vi "Untitled 2.vi"() -> ()   [LabVIEW 2013]
panel:
  out "x 20":dbl
  out "x 19":dbl
  out "x 18":dbl
  out "x 17":dbl
  out "x 16":dbl
  out "x 15":dbl
  out "x 14":dbl
  out "x 13":dbl
  in  "x 12":dbl
  in  "x 11":dbl
  in  "x 10":dbl
  in  "x 9":dbl
  in  "x 8":dbl
  in  "x 7":dbl
  in  "x 6":dbl
  in  "x 5":dbl
  out "x 4":dbl
  in  "x 3":dbl
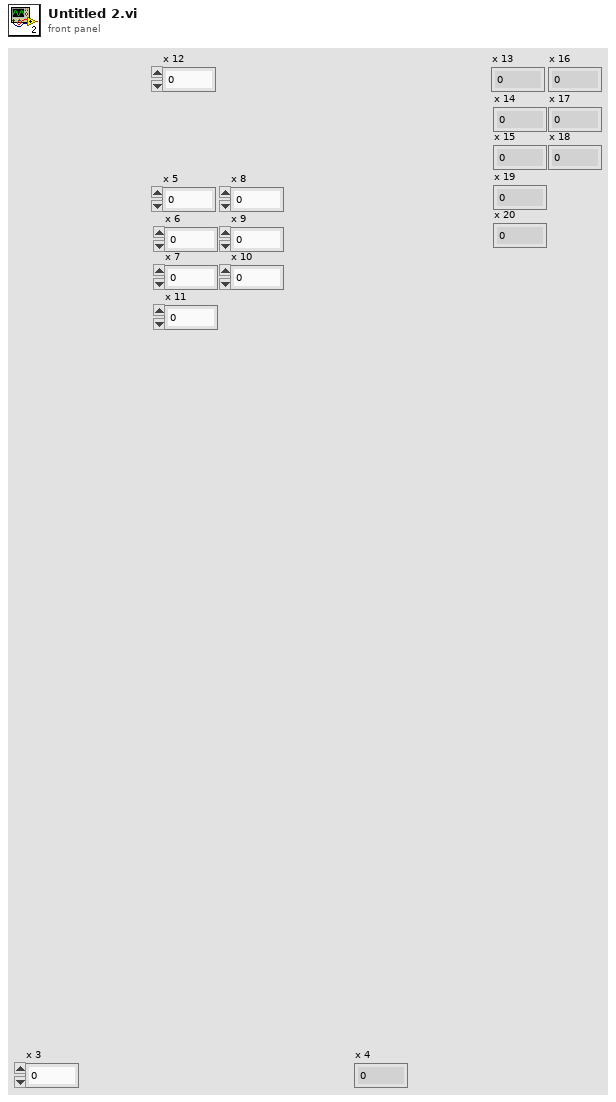
[diagram p1: front panel]
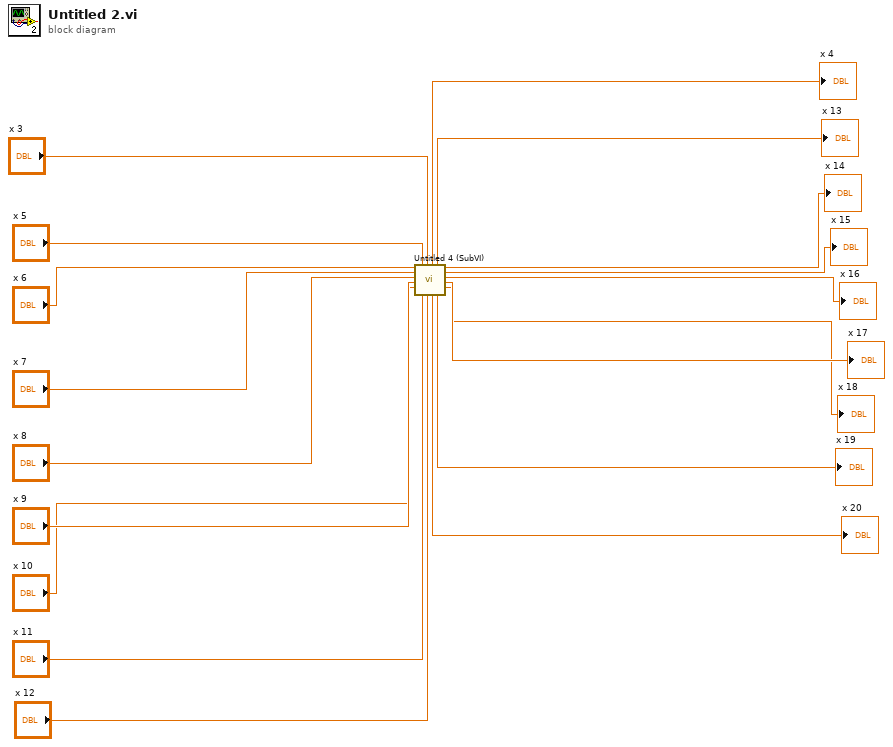
[diagram p0: block diagram]
diagram:
  n1 = call "Untitled 4 (SubVI).vi"("x 19"="x 6", "x 18"="x 7", "x 17"="x 8", "x 16"="x 9", "x 15"="x 10", "x 20"="x 5", "x 14"="x 11", "x 4"="x 3", "x 13"="x 12") -> ("x 3"=→"x 4":dbl, "x 12"=→"x 20":dbl, "x 5"=→"x 13":dbl, "x 11"=→"x 19":dbl, "x 6"=→"x 14":dbl, "x 7"=→"x 15":dbl, "x 8"=→"x 16":dbl, "x 9"=→"x 17":dbl, "x 10"=→"x 18":dbl)  [unwired: 2 in]
